vi "Write Q.vi"(8 "error in (no error)":errorcluster, 10 "Q":dbl, 11 "CRDS Cell in":refnum<class "CRDS Cell.lvclass">) -> (0 "error out":errorcluster, 3 "CRDS Cell out":refnum<class "CRDS Cell.lvclass">)   [LabVIEW 2014, in "CRDS Lib.lvlib" / "CRDS Cell.lvclass"]
uses:
  CRDS Cell.lvclass
  CRDS Cell.lvclass/CRDS Cell.ctl
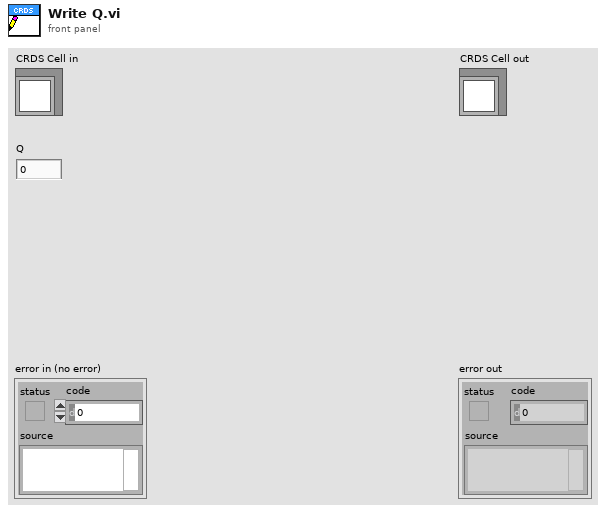
[diagram p1: front panel]
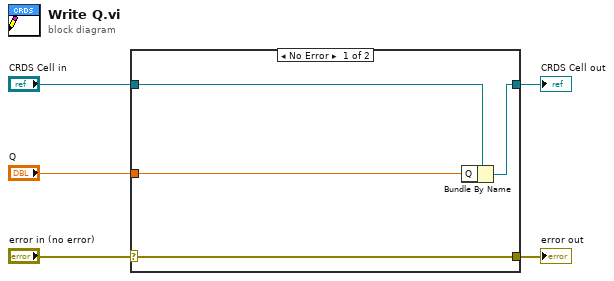
[diagram p0: block diagram]
diagram:
  n1 = case shown="No Error" "error in (no error)" {
    selector: "error in (no error)" -> [w9 w10]
    tunnel: [w9 w10] -> w4
    tunnel: [w7 w11] -> w2
    tunnel: "CRDS Cell in" -> [w8 w11]
    tunnel: "Q" -> [w6 _]
    frame No Error {
      n2 = Bundle By Name(cluster=w8, "Q"=w6) -> (w7:refnum<class "CRDS Cell.lvclass">)
    }
    frame Error {
    }
  }
  "error out" <- w4
  "CRDS Cell out" <- w2
